vi "Receive Dashboard Packet.vi"(7 "connection ID":refnum<k16>) -> ()   [LabVIEW 2015]
uses:
  Common Code/Dashboard Communication/Dashboard Control Data.ctl
  Common Code/Shooter Presets.ctl
  Common Code/Shot Presets.ctl
  Common Code/Encoder Control.ctl
  Common Code/Drivetrain Settings.ctl
  Common Code/Goal Vision Packet.ctl
  Common Code/Dashboard Drivetrain Command.ctl
  Common Code/Drivetrain Vision.ctl
  Common Code/Ball Tracking Command Cluster.ctl
  Common Code/Ball Vision Packet.ctl
  Common Code/Tracking Mode.ctl
  Common Code/Intake Presets.ctl
  Common Code/Drivetrain Output Range.ctl
  Common Code/IntakeEcoderControl.ctl
  Common Code/Climb Presets.ctl
  Common Code/Enabled Systems.ctl
  Common Code/Autonomous Presets.ctl
  Robot Global Data.vi
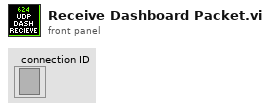
[diagram p1: front panel]
types:
  T1 = typedef "Dashboard Control Data.ctl" = cluster{"Shooter Presets":T2, "Encoder Control":T4, "Steer PID output":cluster{"output high":dbl, "output low":dbl}, " Steer PID gains":cluster{"proportional gain (Kc)":dbl, "integral time (Ti, min)":dbl, "derivative time (Td, min)":dbl}, "Drivetrain Settings":T5, "Vision Packet":T6, "Dashboard Drivetrain Command":T7, "Info/Command Cluster":T9, "Ball Vision Packet":T10, "Intake Presets":T12, "Intake Encoder Control":T14, "Climb Presets":T15, "Goal Output Range":cluster{"output high":dbl, "output low":dbl}, "Enabled Systems":T16, "Auton Presets":T17, "Pressure M":dbl, "Pressure B":dbl, "Vision Timeout":dbl}
  T2 = typedef "Shooter Presets.ctl" = cluster{"Batter Shot":T3, "Deep Middle":T3, "Manual Shot":T3, "Left Ticks Per Rotation":dbl, "Right Ticks Per Rotation":dbl, "Low Bar Shot":T3, "Shooter RPM Tolerance":dbl, "Trigger Power":dbl, "Fire from Load Delay":i32, "Max Angle":dbl, "Min Angle":dbl, "Angle PID gains":cluster{"P":dbl, "I":dbl, "D":dbl}, "Angle Output":cluster{"output high":dbl, "output low":dbl}, "Shooter Angle Tolerance":dbl, "Vision Shoot x^2":dbl, "Vision Shoot x":dbl, "Feed Forward Max Accel":dbl, "Feed Forward Kv":dbl, "Backwards Trigger":dbl, "Shot Finish Delay (ms)":dbl, "Angle Max Current":dbl, "Angle Current Trip Time":dbl, "Intake Angle":dbl, "Vision Shoot c":dbl, "Reset?":bool, "Button Release Delay":dbl, "Angle Pot x":dbl, "Angle Pot c":dbl, "Ignore Angle?":bool, "Max RPM":dbl, "Safty Frist Angle":dbl, "Intake Danger Height":dbl, "Angle Pot B":i32, "Angle Pot M":dbl, "FF Finish RPM":dbl, "RPM PID Right":cluster{"P":dbl, "I":dbl, "D":dbl, "FF":dbl}, "RPM PID Left":cluster{"P":dbl, "I":dbl, "D":dbl, "FF":dbl}, "Backwards RPM":dbl, "Vision RPM":dbl, "Run Wheels Backward Delay":u32, "Cleat Shot":T3}
  T3 = typedef "Shot Presets.ctl" = cluster{"L":dbl, "R":dbl, "A":dbl}
  T4 = typedef "Encoder Control.ctl" = cluster{"Right Tick Constant":dbl, "Left Tick Constant":dbl, "Reset?":bool, "Y Dist":cluster{"PID gains":cluster{"proportional gain (Kc)":dbl, "integral time (Ti, min)":dbl, "derivative time (Td, min)":dbl}}, "Y Stop Thresh":dbl, "Y Stop Speed":dbl}
  T5 = typedef "Drivetrain Settings.ctl" = cluster{"Gyro Tolerance":dbl, "Throttle Ramp (ms)":dbl, "Kv":dbl, "Ka":dbl, "Feed Forward P":dbl, "Feed Forward D":dbl, "Goal Vision PID gains":cluster{"proportional gain (Kc)":dbl, "integral time (Ti, min)":dbl, "derivative time (Td, min)":dbl}, "Goal Detection Window":dbl, "Creep Rate":dbl, "Vision Throttle Threshold":dbl, "Min Turn Output":dbl, "Left Batter Angle":dbl, "Right Batter Angle":dbl}
  T6 = typedef "Goal Vision Packet.ctl" = cluster{"Distance":dbl, "Center X":dbl, "Center Y":dbl, "Found Target?":bool, "Robot Center":dbl, "Angle":dbl}
  T7 = typedef "Dashboard Drivetrain Command.ctl" = cluster{"Drivetrain Vision":T8}
  T8 = typedef "Drivetrain Vision.ctl" = cluster{"Goal Window":dbl, "Ball Window":dbl}
  T9 = typedef "Ball Tracking Command Cluster.ctl" = cluster{"Distance to Ball":dbl, "Desired Angle":dbl, "Command":enum16{"Turn to Ball", "Turn to Angle", "Get Distance"}, "Pixels from Center":dbl}
  T10 = typedef "Ball Vision Packet.ctl" = cluster{"Ball Detected?":bool, "Distance to Ball":dbl, "Desired Angle":dbl, "Pixels from Center":dbl, "Tracking mode":T11}
  T11 = typedef "Tracking Mode.ctl" = enum16{"Turn to Ball", "Turn to Angle"}
  T12 = typedef "Intake Presets.ctl" = cluster{"Intake Speed":dbl, "Outake Speed":dbl, "Low Height":dbl, "Half Height":dbl, "High Idle Height":dbl, "Angle Speed":dbl, "Angle Tolerance":dbl, "Encoder Scale":dbl, "Load Height":dbl, "Output Range":T13, "Rotation Power Max/Min":dbl, "MaxCurrent":dbl, "Intake Trip Time":dbl, "Idle Height":dbl, "Max Height":dbl, "Reset Encoders?":bool, "PID gains":cluster{"proportional gain (Kc)":dbl, "integral time (Ti, min)":dbl, "derivative time (Td, min)":dbl}, "Intake Stop Delay":u32, "Settle Time":dbl, "Settle Wait Time":dbl}
  T13 = typedef "Drivetrain Output Range.ctl" = cluster{"output high":dbl, "output low":dbl}
  T14 = typedef "IntakeEcoderControl.ctl" = cluster{"Arm Tick Constant":dbl, "Reset?":bool, "Y Dist":cluster{"PID gains":cluster{"proportional gain (Kc)":dbl, "integral time (Ti, min)":dbl, "derivative time (Td, min)":dbl}}, "Y Stop Thresh":dbl, "Y Stop Speed":dbl}
  T15 = typedef "Climb Presets.ctl" = cluster{"Pull Power":dbl, "Extend Power":dbl}
  T16 = typedef "Enabled Systems.ctl" = cluster{"Shoot":bool, "Intake":bool, "DT":bool, "Gyro":bool, "100ms":bool, "US":bool}
  T17 = typedef "Autonomous Presets.ctl" = cluster{"Pitch Limit":dbl, "Roll Limit":dbl, "Start Position":dbl, "Cross Position":dbl}
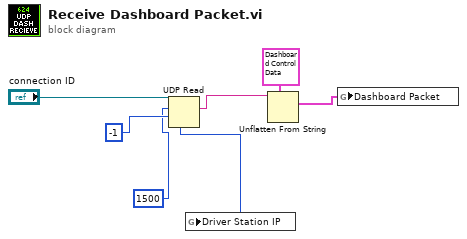
[diagram p0: block diagram]
diagram:
  n1 = UDP Read(connection ID="connection ID", max size (548)=1500, timeout ms (25000)=-1) -> (data out=w4:string, 6:w3:u32)  [unwired: 1 in, 3 out]
  n2 = global write "Robot Global Data.vi" "Driver Station IP"(w3) -> ()
  n3 = Unflatten From String(type=T1 {"Shooter Presets"={"Batter Shot"={"L"=0.0, "R"=0.0, "A"=0.0}, "Deep Middle"={"L"=0.0, "R"=0.0, "A"=0.0}, "Manual Shot"={"L"=0.0, "R"=0.0, "A"=0.0}, "Left Ticks Per Rotation"=0.0, "Right Ticks Per Rotation"=0.0, "Low Bar Shot"={"L"=0.0, "R"=0.0, "A"=0.0}, "Shooter RPM Tolerance"=0.0, "Trigger Power"=0.0, "Fire from Load Delay"=0, "Max Angle"=0.0, "Min Angle"=0.0, "Angle PID gains"={"P"=0.0, "I"=0.0, "D"=0.0}, "Angle Output"={"output high"=0.0, "output low"=0.0}, "Shooter Angle Tolerance"=0.0, "Vision Shoot x^2"=0.0, "Vision Shoot x"=0.0, "Feed Forward Max Accel"=0.0, "Feed Forward Kv"=0.0, "Backwards Trigger"=0.0, "Shot Finish Delay (ms)"=0.0, "Angle Max Current"=0.0, "Angle Current Trip Time"=0.0, "Intake Angle"=0.0, "Vision Shoot c"=0.0, "Reset?"=FALSE, "Button Release Delay"=0.0, "Angle Pot x"=0.0, "Angle Pot c"=0.0, "Ignore Angle?"=FALSE, "Max RPM"=0.0, "Safty Frist Angle"=0.0, "Intake Danger Height"=0.0, "Angle Pot B"=0, "Angle Pot M"=0.0, "FF Finish RPM"=0.0, "RPM PID Right"={"P"=1.0, "I"=0.01, "D"=0.0, "FF"=0.0}, "RPM PID Left"={"P"=1.0, "I"=0.01, "D"=0.0, "FF"=0.0}, "Backwards RPM"=0.0, "Vision RPM"=0.0, "Run Wheels Backward Delay"=0, "Cleat Shot"={"L"=0.0, "R"=0.0, "A"=0.0}}, "Encoder Control"={"Right Tick Constant"=0.0, "Left Tick Constant"=0.0, "Reset?"=FALSE, "Y Dist"={"PID gains"={"proportional gain (Kc)"=0.0, "integral time (Ti, min)"=0.0, "derivative time (Td, min)"=0.0}}, "Y Stop Thresh"=0.0, "Y Stop Speed"=0.0}, "Steer PID output"={"output high"=0.0, "output low"=0.0}, " Steer PID gains"={"proportional gain (Kc)"=0.0, "integral time (Ti, min)"=0.0, "derivative time (Td, min)"=0.0}, "Drivetrain Settings"={"Gyro Tolerance"=0.0, "Throttle Ramp (ms)"=0.0, "Kv"=0.0, "Ka"=0.0, "Feed Forward P"=0.0, "Feed Forward D"=0.0, "Goal Vision PID gains"={"proportional gain (Kc)"=0.0, "integral time (Ti, min)"=0.0, "derivative time (Td, min)"=0.0}, "Goal Detection Window"=0.0, "Creep Rate"=0.0, "Vision Throttle Threshold"=0.0, "Min Turn Output"=0.0, "Left Batter Angle"=0.0, "Right Batter Angle"=0.0}, "Vision Packet"={"Distance"=0.0, "Center X"=0.0, "Center Y"=0.0, "Found Target?"=FALSE, "Robot Center"=0.0, "Angle"=0.0}, "Dashboard Drivetrain Command"={"Drivetrain Vision"={"Goal Window"=0.0, "Ball Window"=0.0}}, "Info/Command Cluster"={"Distance to Ball"=0.0, "Desired Angle"=0.0, "Command"=enum."Turn to Ball", "Pixels from Center"=0.0}, "Ball Vision Packet"={"Ball Detected?"=FALSE, "Distance to Ball"=0.0, "Desired Angle"=0.0, "Pixels from Center"=0.0, "Tracking mode"=enum."Turn to Ball"}, "Intake Presets"={"Intake Speed"=0.0, "Outake Speed"=0.0, "Low Height"=0.0, "Half Height"=0.0, "High Idle Height"=0.0, "Angle Speed"=0.0, "Angle Tolerance"=0.0, "Encoder Scale"=0.0, "Load Height"=0.0, "Output Range"={"output high"=0.0, "output low"=0.0}, "Rotation Power Max/Min"=0.0, "MaxCurrent"=0.0, "Intake Trip Time"=0.0, "Idle Height"=0.0, "Max Height"=0.0, "Reset Encoders?"=FALSE, "PID gains"={"proportional gain (Kc)"=0.0, "integral time (Ti, min)"=0.0, "derivative time (Td, min)"=0.0}, "Intake Stop Delay"=0, "Settle Time"=0.0, "Settle Wait Time"=0.0}, "Intake Encoder Control"={"Arm Tick Constant"=0.0, "Reset?"=FALSE, "Y Dist"={"PID gains"={"proportional gain (Kc)"=0.0, "integral time (Ti, min)"=0.0, "derivative time (Td, min)"=0.0}}, "Y Stop Thresh"=0.0, "Y Stop Speed"=0.0}, "Climb Presets"={"Pull Power"=0.0, "Extend Power"=0.0}, "Goal Output Range"={"output high"=0.0, "output low"=0.0}, "Enabled Systems"={"Shoot"=TRUE, "Intake"=TRUE, "DT"=TRUE, "Gyro"=TRUE, "100ms"=TRUE, "US"=TRUE}, "Auton Presets"={"Pitch Limit"=0.0, "Roll Limit"=0.0, "Start Position"=0.0, "Cross Position"=0.0}, "Pressure M"=0.0, "Pressure B"=0.0, "Vision Timeout"=0.0} ("Dashboard Control Data"), binary string=w4) -> (value=w1:T1)  [unwired: 3 in, 2 out]
  n4 = global write "Robot Global Data.vi" "Dashboard Packet"(w1) -> ()
